vi "Log Payload.vi"(7 "Group Name":string, 8 "error in (no error)":errorcluster, 10 "tdms file":refnum<k34>, 11 "DBL Payload in":refnum<class "DBL Payload.lvclass">) -> (0 "error out":errorcluster, 2 "tdms file out":refnum<k34>, 3 "DBL Payload out":refnum<class "DBL Payload.lvclass">)   [LabVIEW 2015, in "DBL Payload.lvclass"]
uses:
  DBL Payload.lvclass
  Payload.lvclass/Payload.ctl
  Read Name.vi
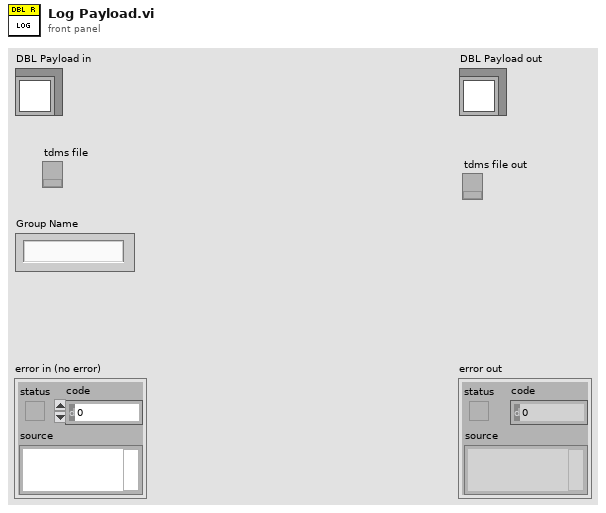
[diagram p1: front panel]
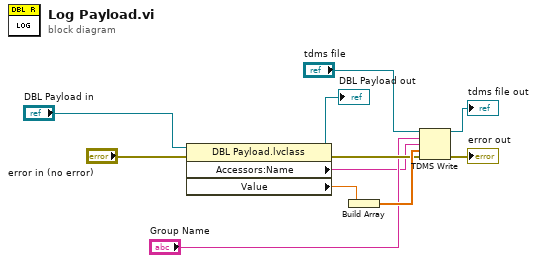
[diagram p0: block diagram]
diagram:
  n1 = property class="DBL Payload.lvclass"(reference="DBL Payload in", error in="error in (no error)") -> (reference out=→"DBL Payload out":refnum<class "DBL Payload.lvclass">, error out=w6:errorcluster, "Accessors:Name"=w1:string, "Value"=w2:dbl)
  n2 = Build Array(w2) -> (w8:dbl[])
  n3 = TDMS Write(0:"tdms file", 5:"Group Name", 7:w1, 9:w8, 11:w6) -> (4:→"tdms file out":refnum<k34>, 15:→"error out":errorcluster)  [unwired: 1 in, 2 out]
